vi "3-5.vi"() -> ()   [LabVIEW 2014]
panel:
  out "?":string
  out "Warning?":bool
  in  "Min Temp.":dbl
  in  "Max Temp.":dbl
  in  "Current Temp.":dbl
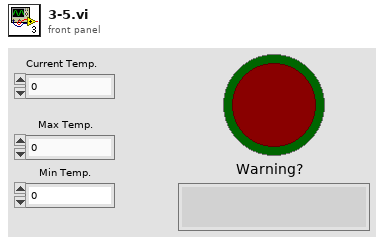
[diagram p1: front panel]
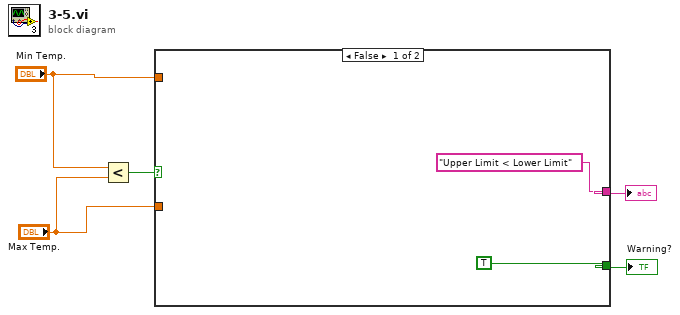
[diagram p0: block diagram]
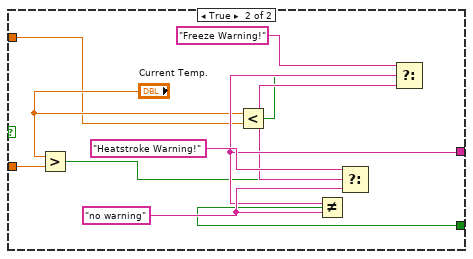
[diagram p2: hidden frame]
diagram:
  n1 = Less?(x="Min Temp.", y="Max Temp.") -> (x < y?=w3:bool)
  n2 = case shown="False" w3 {
    tunnel: [TRUE w17] -> w5
    tunnel: ["Upper Limit < Lower Limit" w14] -> w4
    tunnel: "Max Temp." -> [_ w12]
    tunnel: "Min Temp." -> [_ w9]
    frame False {
    }
    frame True {
      w18 = "no warning"
      n3 = Greater?(x="Current Temp.", y=w12) -> (0:w11:bool)
      n4 = Less?(x="Current Temp.", y=w9) -> (x < y?=w8:bool)
      n5 = Select(t="Heatstroke Warning!", s=w11, f=w18) -> (s? t:f=w13:string)
      n6 = Select(t="Freeze Warning!", s=w8, f=w13) -> (s? t:f=w14:string)
      n7 = Not Equal?(x=w14, y=w18) -> (x != y?=w17:bool)
    }
  }
  "Warning?" <- w5
  "?" <- w4
